vi "Control Arm.vi"(0 "Loop Time (ms)":u32=10, 1 "Arm PID Terms":cluster{"Kp":dbl, "Ki":dbl, "Kd":dbl}={"Kp"=0.00055, "Ki"=0.0, "Kd"=0.0}, 3 "Min Output Arm":dbl=-0.35, 4 "Arm Max Speed to Turn at":dbl=1.0) -> (14 "PID Tracking Arm":T1(graph)={"Goal"=82.91338582677166, "Process Variable"=-0.5174199829351869, "Max Ouput"=0.0, 83.43080580970684, 83.43080580970684, 0.0, -0.0}, 15 "Current Error Arm":dbl=83.43080580970684)   [LabVIEW 2017]
uses:
  <vilib>/Rock Robotics/WPI/ThirdParty/Phoenix-LabVIEW/Motor Controller/Controls/CTRE_Phoenix_MotorControl_ControlMode.ctl
  Globals/Robot Global Data.vi
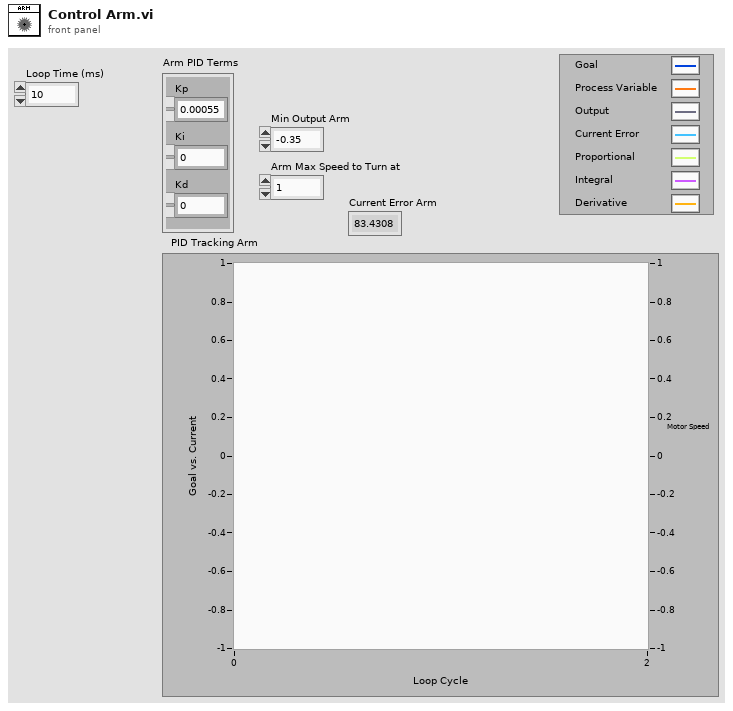
[diagram p1: front panel]
types:
  T1 = cluster{"Goal":dbl, "Process Variable":dbl, "Max Ouput":dbl, dbl, dbl, dbl, dbl}
  T2 = typedef "WPI_MotorControlDeviceRef.ctl" = cluster{"DeviceStatus":errorcluster, "Type":T3, "PWM":cluster{"PWM Channel":T4, "DeadBand":T5}, "CAN":cluster{"Device Number":u8, "SetOutput VI Ref":variant, "GetOutput VI Ref":variant, "Enable VI Ref":variant, "Disable VI Ref":variant, "Data":variant}, "Invert":bool, "DIO PWM":cluster{"PWM \"Enable\" Channel":T4, "DIOChannel":T6, "PWM Rate":dbl}}
  T3 = typedef "WPI_MotorControlType.ctl" = enum16{"PWM", "CAN", "DIO PWM"}
  T4 = typedef "FPGA_DIOPWMChannel.ctl" = enum8{"PWM 0", "PWM 1", "PWM 2", "PWM 3", "PWM 4", "PWM 5", "PWM 6", "PWM 7", "PWM 8", "PWM 9", "PWM MXP 0", "PWM MXP 1", "PWM MXP 2", "PWM MXP 3", "PWM MXP 4", "PWM MXP 5", "PWM MXP 6", "PWM MXP 7", "PWM MXP 8", "PWM MXP 9", "Invalid"}
  T5 = typedef "WPI_PWMDeadband.ctl" = cluster{"Name":string, "maxPositivePwm":i32, "minPositivePwm":i32, "centerPwm":i32, "maxNegativePwm":i32, "minNegativePwm":i32, "angularRange":u16}
  T6 = typedef "FPGA_DIOChannel.ctl" = enum8{"DIO 0", "DIO 1", "DIO 2", "DIO 3", "DIO 4", "DIO 5", "DIO 6", "DIO 7", "DIO 8", "DIO 9", "DIO MXP 0", "DIO MXP 1", "DIO MXP 2", "DIO MXP 3", "DIO MXP 4", "DIO MXP 5", "DIO MXP 6", "DIO MXP 7", "DIO MXP 8", "DIO MXP 9", "DIO MXP 10", "DIO MXP 11", "DIO MXP 12", "DIO MXP 13", "DIO MXP 14", "DIO MXP 15", "SPI Port CS1", "SPI Port CS2", "SPI Port CS3", "SPI Port MISO", "SPI Port MOSI", "Invalid"}
  T7 = typedef "CTRE_Phoenix_MotorControl_ControlMode.ctl" = u16
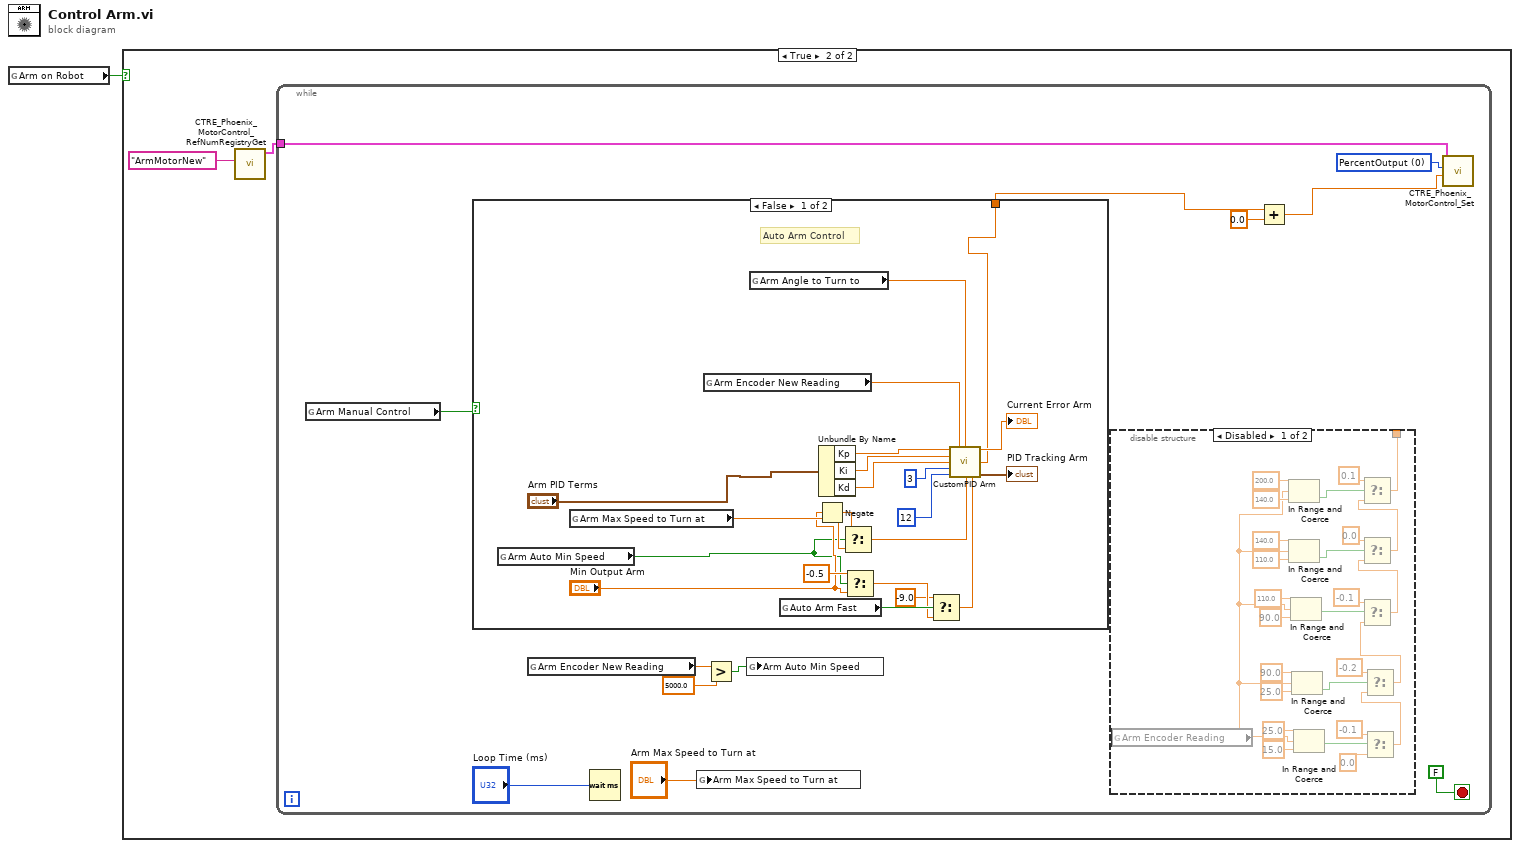
[diagram p0: block diagram]
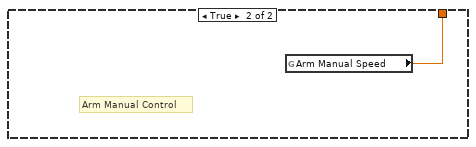
[diagram p4: hidden frame]
diagram:
  n1 = global read "Robot Global Data.vi" "Arm on Robot"() -> (w1:bool)
  n2 = case shown="True" w1 {
    frame False {
    }
    frame True {
      n3 = call "CTRE_Phoenix_MotorControl_RefNumRegistryGet.vi"("refnum name"="ArmMotorNew") -> ("PhoenixMotorControlDevRef"=w2:T2)  [unwired: 9 in, 1 out]
      n4 = while {
        tunnel: w2 -> [w9]
        stop <- FALSE stop-if-true
        w5 = T7 0 items=["PercentOutput"=0, "Position"=1, "Velocity"=2, "Current"=3, "Follower"=5, "MotionProfile"=6, "MotionMagic"=7, "MotionMagicArc"=8, "MotionProfileArc"=10, "Disabled"=15] ("Control Mode")
        n5 = global read "Robot Global Data.vi" "Arm Manual Control"() -> (w12:bool)
        n6 = case shown="False" w12 {
          tunnel: [w55 w64] -> w11
          frame False {
            # "Auto Arm Control"
            n7 = global read "Robot Global Data.vi" "Arm Auto Min Speed"() -> (w47:bool)
            n8 = global read "Robot Global Data.vi" "Arm Max Speed to Turn at"() -> (w51:dbl)
            n9 = global read "Robot Global Data.vi" "Arm Encoder New Reading"() -> (w56:dbl)
            n10 = global read "Robot Global Data.vi" "Arm Angle to Turn to"() -> (w54:dbl)
            n11 = global read "Robot Global Data.vi" "Auto Arm Fast"() -> (w45:bool)
            n12 = Negate(x="Min Output Arm") -> (-x=w49:dbl)
            n13 = Unbundle By Name("Arm PID Terms") -> ("Kp"=w59:dbl, "Ki"=w58:dbl, "Kd"=w57:dbl)
            n14 = Select(t=w49, s=w47, f=w51) -> (s? t:f=w50:dbl)
            n15 = Select(t=-0.5, s=w47, f="Min Output Arm") -> (s? t:f=w44:dbl)
            n16 = Select(t=-9.0, s=w45, f=w44) -> (s? t:f=w46:dbl)
            n17 = call "CustomPID Arm.vi"("Kp"=w59, "Process Variable"=w56, "Goal"=w54, "Ki"=w58, "Kd"=w57, "N-Diff"=3, "N-Int"=12, "Max Ouput"=w50, "Min Output"=w46) -> ("Current Error"=→"Current Error Arm":dbl, "Command"=w55:dbl, "PID Tracking"=→"PID Tracking Arm":T1)  [unwired: 4 in]
          }
          frame True {
            # "Arm Manual Control"
            n18 = global read "Robot Global Data.vi" "Arm Manual Speed"() -> (w64:dbl)
          }
        }
        n19 = global read "Robot Global Data.vi" "Arm Encoder New Reading"() -> (w8:dbl)
        n20 = Wait (ms)(milliseconds to wait="Loop Time (ms)") -> ()  [unwired: 1 out]
        n21 = global write "Robot Global Data.vi" "Arm Max Speed to Turn at"("Arm Max Speed to Turn at") -> ()
        n22 = Greater?(x=w8, y=5000.0) -> (0:w6:bool)
        n23 = global write "Robot Global Data.vi" "Arm Auto Min Speed"(w6) -> ()
        n24 = disable-structure shown="Disabled" {
          disable-tunnel: [w16 _] -> _
          frame Disabled {
            n25 = global read "Robot Global Data.vi" "Arm Encoder Reading"() -> (w17:dbl)
            n26 = In Range and Coerce(upper limit=200.0, x=w17, lower limit=140.0) -> (In Range?=w19:bool)  [unwired: 1 out]
            n27 = In Range and Coerce(upper limit=140.0, x=w17, lower limit=110.0) -> (In Range?=w31:bool)  [unwired: 1 out]
            n28 = In Range and Coerce(upper limit=110.0, x=w17, lower limit=90.0) -> (In Range?=w28:bool)  [unwired: 1 out]
            n29 = In Range and Coerce(upper limit=90.0, x=w17, lower limit=25.0) -> (In Range?=w34:bool)  [unwired: 1 out]
            n30 = In Range and Coerce(upper limit=25.0, x=w17, lower limit=15.0) -> (In Range?=w38:bool)  [unwired: 1 out]
            n31 = Select(t=-0.1, s=w38, f=0.0) -> (s? t:f=w33:dbl)
            n32 = Select(t=-0.2, s=w34, f=w33) -> (s? t:f=w23:dbl)
            n33 = Select(t=-0.1, s=w28, f=w23) -> (s? t:f=w32:dbl)
            n34 = Select(t=0.0, s=w31, f=w32) -> (s? t:f=w18:dbl)
            n35 = Select(t=0.1, s=w19, f=w18) -> (s? t:f=w16:dbl)
          }
          frame Enabled {
          }
        }
        n36 = Add(x=w11, y=0.0) -> (x+y=w4:dbl)
        n37 = call <vilib>:"CTRE_Phoenix_MotorControl_Set.vi"("Output"=w4, "Control Mode"=w5, "PhoenixMotorControlDevRef"=w9) -> ()  [unwired: 7 in, 2 out]
      }
    }
  }
